vi "MT Generate Bits (Galois, Primitive Polynomial).vi"(0 "total bits (128)":i32=128, 7 "specify primitive polynomial":i8[](array[numeric]), 9 "seed in (0xD6BF7DF2)":i32=-692093454 format="%.0x", 11 "error in (no error)":errorcluster, 13 "reset? (T)":bool=TRUE) -> (4 "output bit stream":i8[](array[numeric]), 10 "seed out":i32 format="%.0x", 15 "error out":errorcluster)   [LabVIEW 2020, in "niDMT.lvlib"]
doc: "This polymorphic instance generates Galois pseudonoise (PN) bit sequences. The VI repeats the selected pattern until it generates number of total bits that you specify. Use this instance to specify the primitive polynomial that determines the connection structure of the linear feedback shift register (LFSR)."
uses:
  <vilib>/addons/Modulation/niDMT.lvlib
  <vilib>/addons/Modulation/niAMT.lvlib
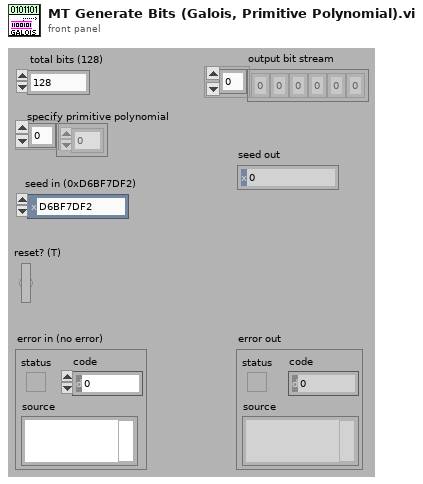
[diagram p1: front panel]
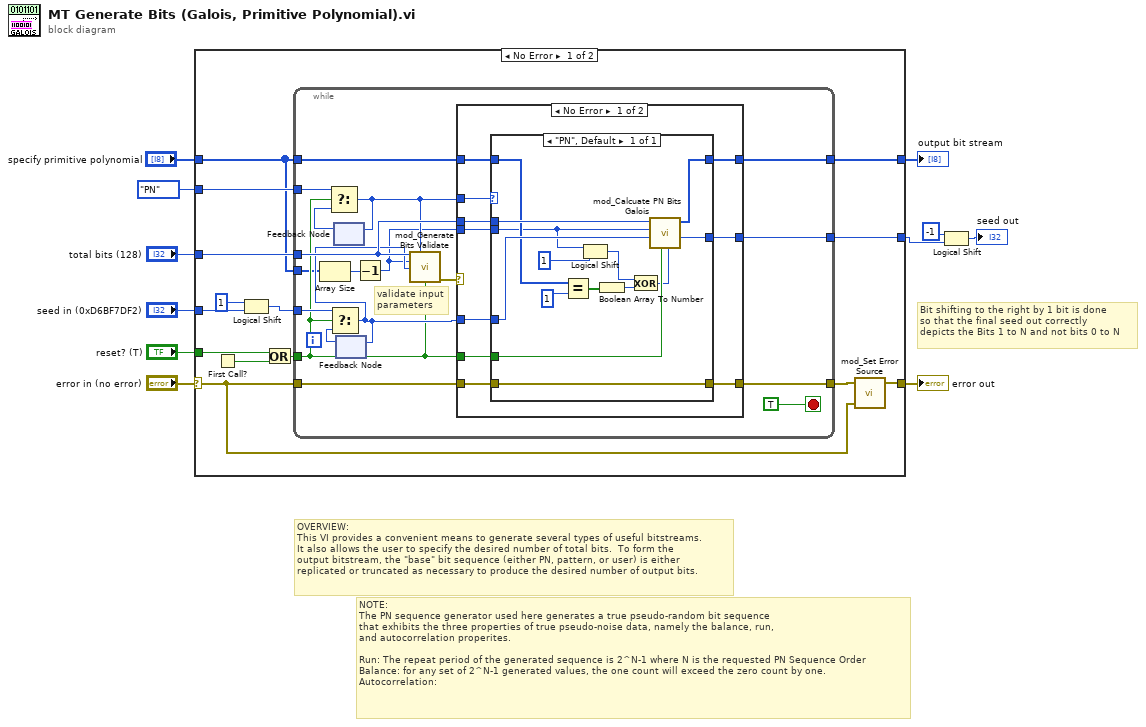
[diagram p0: block diagram]
diagram:
  # "Bit shifting to the right by 1 bit is done \nso that the final seed out correctly \ndepicts the Bits 1 to N and not bits 0 to N"
  # "OVERVIEW:\nThis VI provides a convenient means to generate several types of useful bitstreams.\nIt also allows the user to specify the desired number of total bits.  To form the\noutput bitstream, the \"base\" bit sequence (either PN, pattern, or user) is either\nreplicated or truncated as necessary to produce the desired number of output bits."
  # "NOTE:\nThe PN sequence generator used here generates a true pseudo-random bit sequence\nthat exhibits the three properties of true pseudo-noise data, namely the balance, run,\nand autocorrelation properites.\n\nRun: The repeat period of the generated sequence is 2^N-1 where N is the requested PN Sequence Order\nBalance: for any set of 2^N-1 generated values, the one count will exceed the zero count by one.\nAutocorrelation:"
  n1 = case shown="No Error" "error in (no error)" {
    selector: "error in (no error)" -> [w16 w73]
    tunnel: [w21 w73] -> w10
    tunnel: "total bits (128)" -> [w24 _]
    tunnel: enum16{"PN", "pattern", "user"}."PN" ("mode (PN)") -> [w23 _]
    tunnel: "reset? (T)" -> [w18 _]
    tunnel: "seed in (0xD6BF7DF2)" -> [w13 w72]
    tunnel: [w25 i8[] []] -> w5
    tunnel: [w20 w72] -> w1
    tunnel: "specify primitive polynomial" -> [w15 _]
    frame No Error {
      n2 = First Call?() -> (First Call?: T/F=w19:bool)
      n3 = Logical Shift(y=1, x=w13) -> (x << y=w12:i32)
      n4 = Or(x=w18, y=w19) -> (x .or. y?=w17:bool)
      n5 = while {
        tunnel: [w43] -> w25
        tunnel: w24 -> [w37]
        tunnel: w23 -> [w33]
        tunnel: [w41] -> w22
        tunnel: w16 -> [w40]
        tunnel: [w39] -> w20
        tunnel: w12 -> [w36]
        tunnel: w17 -> [w32]
        tunnel: w15 -> [w29]
        tunnel: w15 -> [w27]
        stop <- TRUE stop-if-true
        # "validate input parameters"
        n6 = Array Size(array=w27) -> (size(s)=w28:i32)
        n7 = feedback #1() -> (w31:enum16{"PN", "pattern", "user"})  [unwired: 1 out]
        n8 = Select(t=w33, s=w32, f=w31) -> (s? t:f=w30:enum16{"PN", "pattern", "user"})
        n9 = feedback-in #1(w30) -> ()
        n10 = feedback #2() -> (w35:i32)  [unwired: 1 out]
        n11 = Select(t=w36, s=w32, f=w35) -> (s? t:f=w34:i32)
        n12 = feedback-in #2(w34) -> ()
        n13 = Decrement(x=w28) -> (x-1=w26:i32)
        n14 = call <vilib>:"mod_Generate Bits Validate.vi"("Total Bits"=w37, "Mode (PN)"=w30, "PN Sequence Order"=w26, "seed in"=w34, "reset?"=w32) -> ("error out"=w42:errorcluster)  [unwired: 1 in, 9 out]
        n15 = case shown="No Error" w42 {
          selector: w42 -> [_ w70]
          tunnel: w40 -> [w53 _]
          tunnel: [w52 w70] -> w41
          tunnel: w30 -> [w51 _]
          tunnel: [w50 i8[] [] ("Output Data Bit Sequence")] -> w43
          tunnel: w37 -> [w49 _]
          tunnel: w34 -> [w48 w69]
          tunnel: w32 -> [w47 _]
          tunnel: [w46 w69] -> w39
          tunnel: w29 -> [w45 _]
          tunnel: w26 -> [w44 _]
          frame No Error {
            n16 = case shown="\"PN\", Default" w51 {
              tunnel: w53 -> [w67]
              tunnel: [w67] -> w52
              tunnel: [w63] -> w50
              tunnel: w49 -> [w62]
              tunnel: w48 -> [w66]
              tunnel: w47 -> [w65]
              tunnel: [w64] -> w46
              tunnel: w45 -> [w58]
              tunnel: w44 -> [w56]
              frame "PN", Default {
                n17 = Equal?(x=w58, y=i8 1) -> (x = y?=w60:bool[])
                n18 = Logical Shift(y=w56, x=u32 1) -> (x << y=w55:u32)
                n19 = Boolean Array To Number(Boolean array=w60) -> (number=w59:u32)
                n20 = Exclusive Or(1:w59, 2:w55) -> (0:w57:u32)
                n21 = call <vilib>:"mod_Calcuate PN Bits Galois.vi"("primitive polynomial coeffs (without MSB)"=w57, "Reset? (T)"=w65, "seed in (0xD6BF7DF2)"=w66, "PN Sequence Order (9)"=w56, "Total Bits"=w62) -> ("seed out"=w64:u32, "Output Bit Stream"=w63:i8[])  [unwired: 5 out]
              }
            }
          }
          frame Error {
            # "Invalid inputs - generate error"
          }
        }
      }
      n22 = call <vilib>:"mod_Set Error Source.vi"("initial error in (no error)"=w16, "final error in (no error)"=w22) -> ("error out"=w21:errorcluster)  [unwired: 3 out]
    }
    frame Error {
    }
  }
  "error out" <- w10
  "output bit stream" <- w5
  n23 = Logical Shift(y=-1, x=w1) -> (x << y=→"seed out":u32)
